vi "Temperature Decline Tester.vi"() -> ()   [LabVIEW 2023]
uses:
  Type Definitions/HEWH Output Information.ctl
  Type Definitions/HEWH Draw Pattern Setup.ctl
  Type Definitions/PRAT Test.ctl
  Utility/Save File/File Setup (Public)/Type Definition/Save File HEWH Heating Control Mode.ctl
  Support VIs/Draw Water Specific/Type Definitions/Terminate Draw Conditions.ctl
  Type Definitions/HEWH Start Conditions.ctl
  Support VIs/Draw Water Specific/Type Definitions/Check Special Condtions.ctl
  Support VIs/Draw Water Specific/Type Definitions/HEWH Special Condition Check.ctl
  Type Definitions/HEWH Draw Flag ENUM.ctl
  Type Definitions/HEWH Specific DAQ.ctl
  Type Definitions/HEWH Power Data.ctl
  Type Definitions/HEWH Power Elements.ctl
  Utility/Type Definitions/UTILITY Power Analyzer.ctl
  Drivers/Viasala Indigo 520/Type Definitions/Viasala Indigo 520 Data.ctl
  Drivers/Tidal Engineering/Type Definitions/Tenney Environmental Chamber Data.ctl
  Type Definitions/HEWH Calc and Calibration.ctl
  Utility/Save File/File Setup (Public)/Type Definition/Save File DOE LabView Program.ctl
  Custom Instrument Control/MW100/Type Definitions/Station ID Selector.ctl
  Range/Type Definitions/RANGE ANSI Rate.ctl
  Custom Instrument Control/MW100/Type Definitions/HEWH Module 4 Relay Status.ctl
  Drivers/Inficon Fusion Micro GC/Type Definitions/Inficon Data.ctl
  Drivers/Alicat Gas Meter Driver/Sub-VIs/Data Cluster.ctl
  Utility/Save File/File Setup.lvlib
panel:
  out "first_iteration":dbl
  out "Run_Timer":dbl
  out "Start Time":dbl
  out "Temp Decline Complete":bool
  in  "Use_Temp_Decline_Method":i16
  in  "Purge_Until_Cutout":i16
  out "prev_cycle_count_out":i32
  out "show_trigger (Debug)":u16
  in  "TC Tree (AVG)":dbl
  in  "stop":bool
  in  "Draw Count":i32
  out "max_temp":dbl
  out "Loop Counter":i32
  out "trigger":u8
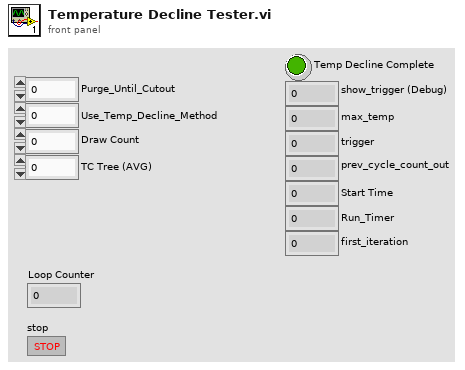
[diagram p1: front panel]
types:
  T1 = typedef "HEWH Output Information.ctl" = cluster{"Scan Rate Adjust":dbl, "Draw Count":i32, "Test Patten Setup":T2, "HEWH Specific DAQ":T10, "Test Output Data":cluster{"PreDraw Data Table":string[][], "Data Table":string[][], "MW100 TC Headers":string[]}, "Calc and Calibration":T16, "Current Draw Time":dbl, "LV Program":T17, "Station ID":T18, "Current Cond":T8, "Test Complete":bool, "ANSI Rate":T19, "Module 4 Relay Status":T20, "Inficon Data Output":T21, "Gas Measurements":cluster{"Gas Measurment Data -Alicat":T22, "Gas Measurment Data - Ritter":cluster{"Gas Flow Rate (L/hr)-Uncorrected":dbl, "Totalized Flow (L)--Uncorrected":dbl, "Gas Flow Rate (cuft/hr)-Uncorrected":dbl, "Totalized Flow (cuft)-Uncorrected":dbl, "Gas Temperature (F)":dbl, "Gas Pressure (in WC)":dbl, "Heise Barometric Pressure (inHG)":dbl, "STP Correction Factor":dbl, "Temp Correction Factor":dbl, "Pressure Correction Factor":dbl, "Water Vapor Pressure":dbl, "Gas Flow Rate (cuft/hr)-Corrected":dbl, "Totalized Flow (cuft)-Corrected":dbl}}}
  T2 = typedef "HEWH Draw Pattern Setup.ctl" = cluster{"Total Gallons Schedule":dbl[], "PRAT/RLT Sequence":T3[], "Current Sequence Index":i32}
  T3 = typedef "PRAT Test.ctl" = cluster{"Sequence #":dbl, "Cycles":i32, "Mode Setting":T4, "Flow Rate (GPM)":dbl, "Temperature (F)":dbl, "Reset Timer":bool, "Use Temp Decline Method":bool, "Terminate Condition":T5, "Condition Value #1":dbl, "UE":bool, "LE":bool, "Comp":bool, "Fan":bool, "Test End Time (Sec)":dbl, "Purge Until Cutout":bool, "Start Conditions":T6, "Condition Value #2":dbl, "Remove Power":bool, "Time":dbl, "Check Special Cond.":T7, "Condition#":T8, "Draw Flags":T9, "Data Processing Delay (FHD 15sec, UEF 5 Sec)":dbl, "Test Complete":bool, "User Setpoint":dbl, "Tank Setpoint":dbl}
  T4 = typedef "File Setup.lvlib/Save File HEWH Heating Control Mode.ctl" = string
  T5 = typedef "Terminate Draw Conditions.ctl" = enum16{"C1-Terminate Draw @ Gallon Mark", "C2-Special Last Draw (HU Test)", "C3-RTD Out <=", "C4-Mean Tank Temp <=", "C5-Decrease RTD Out (Deg F)", "C6-Time (Seconds)", "C7-Until Any Heat Source", "C8-Specific Heat Source", "C9-Do Nothing", "C10-Inlet Outlet RTD Temp Delta"}
  T6 = typedef "HEWH Start Conditions.ctl" = enum16{"Heat Source Cutout", "At Time (Seconds)", "Every X (Seconds)", "T2 >= X° Below Setpoint", "Seconds From Complete", "Wait for LE & Comp Cutout", "Wait for Comp Cutout", "Wait for LE Cutout", "Wait for UE Cutout", "Start Immediately"}
  T7 = typedef "Check Special Condtions.ctl" = enum16{"SC1-Do Nothing", "SC2-Check Heat Source (On-C2/Off-C1)", "SC3-Check Skip Condition", "SC4-Check Heat Source ON/Fail", "SC5-Keep Draw Valves Open", "SC6-Skip Purge"}
  T8 = typedef "HEWH Special Condition Check.ctl" = enum16{"N/A", "C1", "C2", "Reset/Fail", "Skip Draw Sequence"}
  T9 = typedef "HEWH Draw Flag ENUM.ctl" = enum16{"N/A", "None(0)", "Sml(1)", "Med(2)", "SmlMed(3)", "Lrg(4)", "SmlLrg(5)", "MedLrg(6)", "SmlMedLrg(7)"}
  T10 = typedef "HEWH Specific DAQ.ctl" = cluster{"HEWH Data":T11, "Flow Valve % Open":dbl, "Power State":T12, "Power Analyzer":T13, "Flow Valve uA Output":i32, "Gallons Start (Gal)":dbl, "PI Output":dbl, "Viasala Indigo 520 Data":T14, "Tenney Environmental Chamber Data Output":T15}
  T11 = typedef "HEWH Power Data.ctl" = cluster{"HEWH Standard":cluster{"Voltage (Volts)":dbl, "Current (Amps)":dbl, "Power (Watts)":dbl, "WattHours (Wh)":dbl, "TC Tree (AVG)":dbl, "Flow Rate (GPM)":dbl, "Gallons (Gal)":dbl, "RTD Out (Deg F)":dbl, "RTD In (Deg F)":dbl, "RTD Amb (Deg F)":dbl, "TC Down":dbl, "UE Event Lead":i32, "LE Event Lead":i32, "TC 8":dbl, "TC 9":dbl, "TC 10":dbl, "TC Tree Array (1-6)":dbl[], "TC 7":dbl, "PSI 1":dbl, "PSI 2":dbl, "PSI 3":dbl, "PSI 4":dbl, "Gas BTU":dbl, "Gas BTU/hr":dbl}, "PRAT":cluster{"Power (Watts) A":dbl, "Power (Watts) B":dbl, "Power (Watts) C":dbl, "Power (Watts) D":dbl, "TC1":dbl, "TC2":dbl, "TC3":dbl, "TC4":dbl, "WattHours (Wh) A":dbl, "WattHours (Wh) B":dbl, "WattHours (Wh) C":dbl, "WattHours (Wh) D":dbl, "Ambient":dbl, "Extra Temp":dbl}, "Additional Power Data":cluster{"Vthd":dbl, "Frequency (Hz)":dbl, "Apparent Power (VA)":dbl, "Power Factor":dbl, "Current Crest Factor":dbl, "Voltage Crest Factor":dbl, "Integration Time (sec)":dbl}}
  T12 = typedef "HEWH Power Elements.ctl" = cluster{"UE":bool, "LE":bool, "COMP":bool, "FANS":bool}
  T13 = typedef "UTILITY Power Analyzer.ctl" = enum16{"", "APLUS", "WT210", "WT500", "WT300", "OSI", "Debug", "WT230", "WT300_1", "WT300_2"}
  T14 = typedef "Viasala Indigo 520 Data.ctl" = cluster{"Temperature Probe 1":dbl, "Humidity Probe 1":dbl, "Temperature Probe 2":dbl, "Humidity Probe 2":dbl}
  T15 = typedef "Tenney Environmental Chamber Data.ctl" = cluster{"Temperature Setpoint":dbl, "Temperature Process Variable":dbl, "Humidity Setpoint":dbl, "Humidity Process Variable":dbl, "Frequency Setpoint":dbl, "Frequency Process Variable":dbl, "Chamber Status (ON/OFF)":string}
  T16 = typedef "HEWH Calc and Calibration.ctl" = cluster{"Mean SD Var Max Min Array":string[][], "Draw Statistics (DBL)":dbl[][], "Calibration Coefficients DBL":dbl[][], "Start Gallons":dbl, "Starting Temp Decline":dbl, "K-Factor (Temperature)":dbl, "All Draw Stats":string[][], "RTD Terminate Value":dbl, "K-Factor (Flow)":dbl, "Intellifaucet Type":string, "Thermal Stabil Array":dbl[][], "Gas Thermal Stabil Complete":bool, "Therm Reset Cmpt 1":bool, "Therm Reset Cmpt 2":bool, "Last Flow Rate (Therm)":dbl, "State":enum16{"State 0", "State 1", "State 2", "State 3", "State 4", "State 5", "State 6"}, "Gas Thermal Time":dbl, "Target Rate (Thermal)":dbl, "Thermal - Final":dbl[][], "State5 Gal Water":dbl, "State 5 Gal Gas":dbl, "Intellif Open < 1":dbl, "Intellif Open < 1.7":dbl, "Intellif Open < 2.2":dbl, "Intellif Open > 2.2":dbl, "End of Draw\nComparison":bool[][], "Temperature Decline Method":cluster{"Previous Cycle Count":i32, "Previous Max Temp In":dbl, "Previous Trigger In":u8, "Start Timer":dbl, "first_iteration":dbl}}
  T17 = typedef "File Setup.lvlib/Save File DOE LabView Program.ctl" = enum16{"No Name Found", "DOE Stand", "Dishwasher Kitchen", "Portable Stand", "HEWH", "Dryer", "Dryer WILT", "HCC", "PRAT", "HEWH RLT", "Refrigeration", "Gas Water Heater"}
  T18 = typedef "Station ID Selector.ctl" = enum16{"", "A", "B", "C", "D", "Global"}
  T19 = typedef "RANGE ANSI Rate.ctl" = cluster{"Array 1":dbl[], "Array 3":dbl[], "Array 2":dbl[], "Start ANSI":bool, "ANSI Start Time":dbl, "Restart ANSI":bool, "15 Min ANSI Avg (BTU/hr)":dbl, "20 Min ANSI Avg (BTU/hr)":dbl, "25 Min ANSI Avg (BTU/hr)":dbl, "Absolute Pressure":dbl, "Gas Temperature":dbl, "Volumetric Flow Rate":dbl, "Mass Flow Rate":dbl, "Array 4":dbl[], "Array 5":dbl[], "Gas Rate":dbl, "15 Min Pres Avg (PSIA)":dbl, "20 Min Pres Avg (PSIA)":dbl, "25 Min Pres Avg (PSIA)":dbl, "15 Min Temp Avg (°F) ":dbl, "20 Min Temp Avg (°F)":dbl, "25 Min Temp Avg (°F)":dbl, "15 Min Uncorrected Avg (CFH)":dbl, "20 Min Uncorrected Avg (CFH)":dbl, "25 Min Uncorrected Avg (CFH)":dbl, "15 Min Corrected Avg (SCFH)":dbl, "20 Min Corrected Avg (SCFH)":dbl, "25 Min Corrected Avg (SCFH)":dbl, "15 Min Complete":bool, "20 Min Complete":bool, "25 Min Complete":bool, "Heating Value (BTU/ft³)":dbl, "CO CO2 15 Min":string[][], "CO CO2 20 Min":string[][], "CO CO2 25 Min":string[][], "CO CO2 Real Time":string[][]}
  T20 = typedef "HEWH Module 4 Relay Status.ctl" = cluster{"INTELLIFAUCET TEMP(T)/FLOW(F) (CH 041)":bool, "INTELLIFAUCET READY (CH 042)":bool, "INTELLIFAUCET START (CH 043)":bool, "INTELLIFAUCET STOP (CH 044)":bool, "MAIN POWER RELAY (CH 047)":bool, "NOT USED (CH 045)":bool, "NOT USED (CH 046)":bool, "PURGE VALVE RELAY (CH 048)":bool, "OUTLET VALVE RELAY (CH 049)":bool, "INLET VALVE RELAY (CH 050)":bool, "Intellifaucet (% Open)":dbl, "Proportioning Valve (%Open)":dbl, "Intellifaucet Temp Setpoint (F)":dbl}
  T21 = typedef "Inficon Data.ctl" = cluster{"Gross Heating Value, Vol (Real, Dry)":dbl, "Nitrogen Component Normalized Mole % (Dry)":dbl, "Methane Component Normalized Mole % (Dry)":dbl, "Carbon Dioxide Component Normalized Mole % (Dry)":dbl, "Ethane Component Normalized Mole % (Dry)":dbl, "Propane Component Normalized Mole % (Dry)":dbl, "i-Pentane Component Normalized Mole % (Dry)":dbl, "i-Butane Component Normalized Mole % (Dry)":dbl, "n-Butane Component Normalized Mole % (Dry)":dbl, "n-Pentane Component Normalized Mole % (Dry)":dbl, "Hexane Component Normalized Mole % (Dry)":dbl, "Heptane Component Normalized Mole % (Dry)":dbl, "Gross Wobbe Index, Real(Dry)":dbl, "Relative Density, Real(Dry)":dbl, "Propylene Component Normalized Mole % (Dry)":dbl, "C4 Olefins Component Normalized Mole % (Dry)":dbl, "Water Component Normalized Mole % (Dry)":dbl, "Gross Heating Value, Vol (Real, Sat)":dbl}
  T22 = typedef "Data Cluster.ctl" = cluster{"Absolute Pressure":dbl, "Gauge/Diff. Pressure":dbl, "Barometric Pressure":dbl, "Temperature":dbl, "Volumetric Flow":dbl, "Mass Flow":dbl, "Setpoint":dbl, "Valve Drive":dbl, "Totalizer":dbl, "[hr]":dbl, "[min]":dbl, "[sec]":dbl, "Totalizer Average Flow":dbl, "Totalizer Peak Flow":dbl, "Gas selected":string}
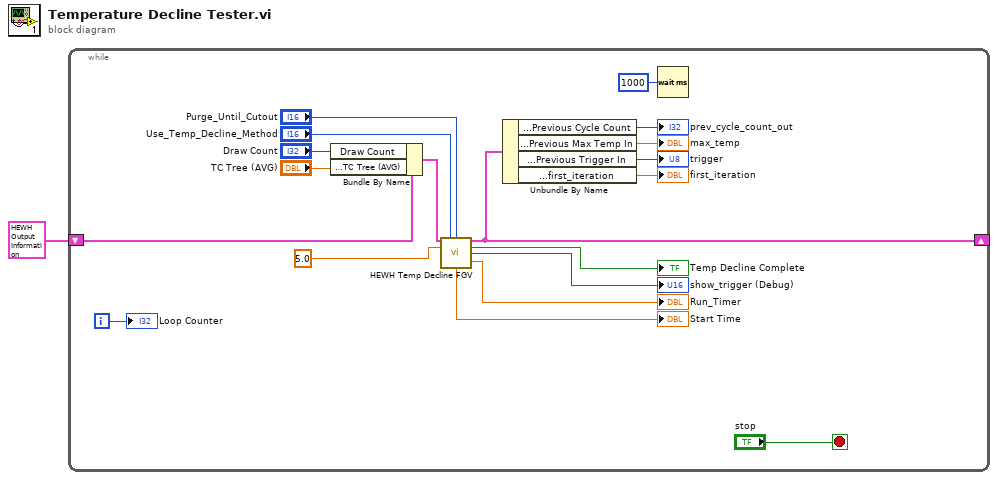
[diagram p0: block diagram]
diagram:
  n1 = while {
    shift-right: [w11] -> _
    shift-left: T1 {"Scan Rate Adjust"=0.0, "Draw Count"=0, "Test Patten Setup"={"Total Gallons Schedule"=[], "PRAT/RLT Sequence"=[{"Sequence #"=1.0, "Cycles"=35, "Mode Setting"="", "Flow Rate (GPM)"=0.0, "Temperature (F)"=0.0, "Reset Timer"=FALSE, "Use Temp Decline Method"=FALSE, "Terminate Condition"=enum."C1-Terminate Draw @ Gallon Mark", "Condition Value #1"=0.0, "UE"=FALSE, "LE"=FALSE, "Comp"=FALSE, "Fan"=FALSE, "Test End Time (Sec)"=0.0, "Purge Until Cutout"=FALSE, "Start Conditions"=enum."Heat Source Cutout", "Condition Value #2"=0.0, "Remove Power"=FALSE, "Time"=0.0, "Check Special Cond."=enum."SC1-Do Nothing", "Condition#"=enum."C1", "Draw Flags"=enum."N/A", "Data Processing Delay (FHD 15sec, UEF 5 Sec)"=0.0, "Test Complete"=FALSE, "User Setpoint"=0.0, "Tank Setpoint"=0.0}, {"Sequence #"=2.0, "Cycles"=15, "Mode Setting"="", "Flow Rate (GPM)"=0.0, "Temperature (F)"=0.0, "Reset Timer"=FALSE, "Use Temp Decline Method"=FALSE, "Terminate Condition"=enum."C1-Terminate Draw @ Gallon Mark", "Condition Value #1"=0.0, "UE"=FALSE, "LE"=FALSE, "Comp"=FALSE, "Fan"=FALSE, "Test End Time (Sec)"=0.0, "Purge Until Cutout"=FALSE, "Start Conditions"=enum."Heat Source Cutout", "Condition Value #2"=0.0, "Remove Power"=FALSE, "Time"=0.0, "Check Special Cond."=enum."SC1-Do Nothing", "Condition#"=enum."C1", "Draw Flags"=enum."N/A", "Data Processing Delay (FHD 15sec, UEF 5 Sec)"=0.0, "Test Complete"=FALSE, "User Setpoint"=0.0, "Tank Setpoint"=0.0}, {"Sequence #"=3.0, "Cycles"=35, "Mode Setting"="", "Flow Rate (GPM)"=0.0, "Temperature (F)"=0.0, "Reset Timer"=FALSE, "Use Temp Decline Method"=FALSE, "Terminate Condition"=enum."C1-Terminate Draw @ Gallon Mark", "Condition Value #1"=0.0, "UE"=FALSE, "LE"=FALSE, "Comp"=FALSE, "Fan"=FALSE, "Test End Time (Sec)"=0.0, "Purge Until Cutout"=FALSE, "Start Conditions"=enum."Heat Source Cutout", "Condition Value #2"=0.0, "Remove Power"=FALSE, "Time"=0.0, "Check Special Cond."=enum."SC1-Do Nothing", "Condition#"=enum."C1", "Draw Flags"=enum."N/A", "Data Processing Delay (FHD 15sec, UEF 5 Sec)"=0.0, "Test Complete"=FALSE, "User Setpoint"=0.0, "Tank Setpoint"=0.0}, {"Sequence #"=4.0, "Cycles"=15, "Mode Setting"="", "Flow Rate (GPM)"=0.0, "Temperature (F)"=0.0, "Reset Timer"=FALSE, "Use Temp Decline Method"=FALSE, "Terminate Condition"=enum."C1-Terminate Draw @ Gallon Mark", "Condition Value #1"=0.0, "UE"=FALSE, "LE"=FALSE, "Comp"=FALSE, "Fan"=FALSE, "Test End Time (Sec)"=0.0, "Purge Until Cutout"=FALSE, "Start Conditions"=enum."Heat Source Cutout", "Condition Value #2"=0.0, "Remove Power"=FALSE, "Time"=0.0, "Check Special Cond."=enum."SC1-Do Nothing", "Condition#"=enum."C1", "Draw Flags"=enum."N/A", "Data Processing Delay (FHD 15sec, UEF 5 Sec)"=0.0, "Test Complete"=FALSE, "User Setpoint"=0.0, "Tank Setpoint"=0.0}, {"Sequence #"=5.0, "Cycles"=35, "Mode Setting"="", "Flow Rate (GPM)"=0.0, "Temperature (F)"=0.0, "Reset Timer"=FALSE, "Use Temp Decline Method"=FALSE, "Terminate Condition"=enum."C1-Terminate Draw @ Gallon Mark", "Condition Value #1"=0.0, "UE"=FALSE, "LE"=FALSE, "Comp"=FALSE, "Fan"=FALSE, "Test End Time (Sec)"=0.0, "Purge Until Cutout"=FALSE, "Start Conditions"=enum."Heat Source Cutout", "Condition Value #2"=0.0, "Remove Power"=FALSE, "Time"=0.0, "Check Special Cond."=enum."SC1-Do Nothing", "Condition#"=enum."C1", "Draw Flags"=enum."N/A", "Data Processing Delay (FHD 15sec, UEF 5 Sec)"=0.0, "Test Complete"=FALSE, "User Setpoint"=0.0, "Tank Setpoint"=0.0}, {"Sequence #"=6.0, "Cycles"=15, "Mode Setting"="", "Flow Rate (GPM)"=0.0, "Temperature (F)"=0.0, "Reset Timer"=FALSE, "Use Temp Decline Method"=FALSE, "Terminate Condition"=enum."C1-Terminate Draw @ Gallon Mark", "Condition Value #1"=0.0, "UE"=FALSE, "LE"=FALSE, "Comp"=FALSE, "Fan"=FALSE, "Test End Time (Sec)"=0.0, "Purge Until Cutout"=FALSE, "Start Conditions"=enum."Heat Source Cutout", "Condition Value #2"=0.0, "Remove Power"=FALSE, "Time"=0.0, "Check Special Cond."=enum."SC1-Do Nothing", "Condition#"=enum."C1", "Draw Flags"=enum."N/A", "Data Processing Delay (FHD 15sec, UEF 5 Sec)"=0.0, "Test Complete"=FALSE, "User Setpoint"=0.0, "Tank Setpoint"=0.0}, {"Sequence #"=7.0, "Cycles"=35, "Mode Setting"="", "Flow Rate (GPM)"=0.0, "Temperature (F)"=0.0, "Reset Timer"=FALSE, "Use Temp Decline Method"=FALSE, "Terminate Condition"=enum."C1-Terminate Draw @ Gallon Mark", "Condition Value #1"=0.0, "UE"=FALSE, "LE"=FALSE, "Comp"=FALSE, "Fan"=FALSE, "Test End Time (Sec)"=0.0, "Purge Until Cutout"=FALSE, "Start Conditions"=enum."Heat Source Cutout", "Condition Value #2"=0.0, "Remove Power"=FALSE, "Time"=0.0, "Check Special Cond."=enum."SC1-Do Nothing", "Condition#"=enum."C1", "Draw Flags"=enum."N/A", "Data Processing Delay (FHD 15sec, UEF 5 Sec)"=0.0, "Test Complete"=FALSE, "User Setpoint"=0.0, "Tank Setpoint"=0.0}, {"Sequence #"=8.0, "Cycles"=15, "Mode Setting"="", "Flow Rate (GPM)"=0.0, "Temperature (F)"=0.0, "Reset Timer"=FALSE, "Use Temp Decline Method"=FALSE, "Terminate Condition"=enum."C1-Terminate Draw @ Gallon Mark", "Condition Value #1"=0.0, "UE"=FALSE, "LE"=FALSE, "Comp"=FALSE, "Fan"=FALSE, "Test End Time (Sec)"=0.0, "Purge Until Cutout"=FALSE, "Start Conditions"=enum."Heat Source Cutout", "Condition Value #2"=0.0, "Remove Power"=FALSE, "Time"=0.0, "Check Special Cond."=enum."SC1-Do Nothing", "Condition#"=enum."C1", "Draw Flags"=enum."N/A", "Data Processing Delay (FHD 15sec, UEF 5 Sec)"=0.0, "Test Complete"=FALSE, "User Setpoint"=0.0, "Tank Setpoint"=0.0}], "Current Sequence Index"=0}, "HEWH Specific DAQ"={"HEWH Data"={"HEWH Standard"={"Voltage (Volts)"=0.0, "Current (Amps)"=0.0, "Power (Watts)"=0.0, "WattHours (Wh)"=0.0, "TC Tree (AVG)"=0.0, "Flow Rate (GPM)"=0.0, "Gallons (Gal)"=0.0, "RTD Out (Deg F)"=0.0, "RTD In (Deg F)"=0.0, "RTD Amb (Deg F)"=0.0, "TC Down"=0.0, "UE Event Lead"=0, "LE Event Lead"=0, "TC 8"=0.0, "TC 9"=0.0, "TC 10"=0.0, "TC Tree Array (1-6)"=[], "TC 7"=0.0, "PSI 1"=0.0, "PSI 2"=0.0, "PSI 3"=0.0, "PSI 4"=0.0, "Gas BTU"=0.0, "Gas BTU/hr"=0.0}, "PRAT"={"Power (Watts) A"=0.0, "Power (Watts) B"=0.0, "Power (Watts) C"=0.0, "Power (Watts) D"=0.0, "TC1"=0.0, "TC2"=0.0, "TC3"=0.0, "TC4"=0.0, "WattHours (Wh) A"=0.0, "WattHours (Wh) B"=0.0, "WattHours (Wh) C"=0.0, "WattHours (Wh) D"=0.0, "Ambient"=0.0, "Extra Temp"=0.0}, "Additional Power Data"={"Vthd"=0.0, "Frequency (Hz)"=0.0, "Apparent Power (VA)"=0.0, "Power Factor"=0.0, "Current Crest Factor"=0.0, "Voltage Crest Factor"=0.0, "Integration Time (sec)"=0.0}}, "Flow Valve % Open"=0.0, "Power State"={"UE"=FALSE, "LE"=FALSE, "COMP"=FALSE, "FANS"=FALSE}, "Power Analyzer"=enum."APLUS", "Flow Valve uA Output"=0, "Gallons Start (Gal)"=0.0, "PI Output"=0.0, "Viasala Indigo 520 Data"={"Temperature Probe 1"=0.0, "Humidity Probe 1"=0.0, "Temperature Probe 2"=0.0, "Humidity Probe 2"=0.0}, "Tenney Environmental Chamber Data Output"={"Temperature Setpoint"=0.0, "Temperature Process Variable"=0.0, "Humidity Setpoint"=0.0, "Humidity Process Variable"=0.0, "Frequency Setpoint"=0.0, "Frequency Process Variable"=0.0, "Chamber Status (ON/OFF)"=""}}, "Test Output Data"={"PreDraw Data Table"=[], "Data Table"=[], "MW100 TC Headers"=[]}, "Calc and Calibration"={"Mean SD Var Max Min Array"=[], "Draw Statistics (DBL)"=[], "Calibration Coefficients DBL"=[], "Start Gallons"=0.0, "Starting Temp Decline"=0.0, "K-Factor (Temperature)"=0.0, "All Draw Stats"=[], "RTD Terminate Value"=0.0, "K-Factor (Flow)"=0.0, "Intellifaucet Type"="", "Thermal Stabil Array"=[], "Gas Thermal Stabil Complete"=FALSE, "Therm Reset Cmpt 1"=FALSE, "Therm Reset Cmpt 2"=FALSE, "Last Flow Rate (Therm)"=0.0, "State"=enum."State 1", "Gas Thermal Time"=0.0, "Target Rate (Thermal)"=0.0, "Thermal - Final"=[], "State5 Gal Water"=0.0, "State 5 Gal Gas"=0.0, "Intellif Open < 1"=0.0, "Intellif Open < 1.7"=0.0, "Intellif Open < 2.2"=0.0, "Intellif Open > 2.2"=0.0, "End of Draw\nComparison"=[], "Temperature Decline Method"={"Previous Cycle Count"=0, "Previous Max Temp In"=0.0, "Previous Trigger In"=0, "Start Timer"=0.0, "first_iteration"=0.0}}, "Current Draw Time"=0.0, "LV Program"=enum."HEWH", "Station ID"=enum."A", "Current Cond"=enum."N/A", "Test Complete"=FALSE, "ANSI Rate"={"Array 1"=[], "Array 3"=[], "Array 2"=[], "Start ANSI"=FALSE, "ANSI Start Time"=0.0, "Restart ANSI"=FALSE, "15 Min ANSI Avg (BTU/hr)"=0.0, "20 Min ANSI Avg (BTU/hr)"=0.0, "25 Min ANSI Avg (BTU/hr)"=0.0, "Absolute Pressure"=0.0, "Gas Temperature"=0.0, "Volumetric Flow Rate"=0.0, "Mass Flow Rate"=0.0, "Array 4"=[], "Array 5"=[], "Gas Rate"=0.0, "15 Min Pres Avg (PSIA)"=0.0, "20 Min Pres Avg (PSIA)"=0.0, "25 Min Pres Avg (PSIA)"=0.0, "15 Min Temp Avg (°F) "=0.0, "20 Min Temp Avg (°F)"=0.0, "25 Min Temp Avg (°F)"=0.0, "15 Min Uncorrected Avg (CFH)"=0.0, "20 Min Uncorrected Avg (CFH)"=0.0, "25 Min Uncorrected Avg (CFH)"=0.0, "15 Min Corrected Avg (SCFH)"=0.0, "20 Min Corrected Avg (SCFH)"=0.0, "25 Min Corrected Avg (SCFH)"=0.0, "15 Min Complete"=FALSE, "20 Min Complete"=FALSE, "25 Min Complete"=FALSE, "Heating Value (BTU/ft³)"=0.0, "CO CO2 15 Min"=[], "CO CO2 20 Min"=[], "CO CO2 25 Min"=[], "CO CO2 Real Time"=[]}, "Module 4 Relay Status"={"INTELLIFAUCET TEMP(T)/FLOW(F) (CH 041)"=FALSE, "INTELLIFAUCET READY (CH 042)"=FALSE, "INTELLIFAUCET START (CH 043)"=FALSE, "INTELLIFAUCET STOP (CH 044)"=FALSE, "MAIN POWER RELAY (CH 047)"=FALSE, "NOT USED (CH 045)"=FALSE, "NOT USED (CH 046)"=FALSE, "PURGE VALVE RELAY (CH 048)"=FALSE, "OUTLET VALVE RELAY (CH 049)"=FALSE, "INLET VALVE RELAY (CH 050)"=FALSE, "Intellifaucet (% Open)"=0.0, "Proportioning Valve (%Open)"=0.0, "Intellifaucet Temp Setpoint (F)"=0.0}, "Inficon Data Output"={"Gross Heating Value, Vol (Real, Dry)"=1067.4462890625, "Nitrogen Component Normalized Mole % (Dry)"=0.0, "Methane Component Normalized Mole % (Dry)"=92.87550354003906, "Carbon Dioxide Component Normalized Mole % (Dry)"=0.1941000074148178, "Ethane Component Normalized Mole % (Dry)"=6.454999923706055, "Propane Component Normalized Mole % (Dry)"=0.3865000009536743, "i-Pentane Component Normalized Mole % (Dry)"=0.007799999788403511, "i-Butane Component Normalized Mole % (Dry)"=0.03880000114440918, "n-Butane Component Normalized Mole % (Dry)"=0.03819999843835831, "n-Pentane Component Normalized Mole % (Dry)"=0.004100000020116568, "Hexane Component Normalized Mole % (Dry)"=0.0, "Heptane Component Normalized Mole % (Dry)"=0.0, "Gross Wobbe Index, Real(Dry)"=1385.8905029296875, "Relative Density, Real(Dry)"=0.5932452082633972, "Propylene Component Normalized Mole % (Dry)"=0.0, "C4 Olefins Component Normalized Mole % (Dry)"=0.0, "Water Component Normalized Mole % (Dry)"=0.0, "Gross Heating Value, Vol (Real, Sat)"=0.0}, "Gas Measurements"={"Gas Measurment Data -Alicat"={"Absolute Pressure"=0.0, "Gauge/Diff. Pressure"=0.0, "Barometric Pressure"=0.0, "Temperature"=0.0, "Volumetric Flow"=0.0, "Mass Flow"=0.0, "Setpoint"=0.0, "Valve Drive"=0.0, "Totalizer"=0.0, "[hr]"=0.0, "[min]"=0.0, "[sec]"=0.0, "Totalizer Average Flow"=0.0, "Totalizer Peak Flow"=0.0, "Gas selected"=""}, "Gas Measurment Data - Ritter"={"Gas Flow Rate (L/hr)-Uncorrected"=0.0, "Totalized Flow (L)--Uncorrected"=0.0, "Gas Flow Rate (cuft/hr)-Uncorrected"=0.0, "Totalized Flow (cuft)-Uncorrected"=0.0, "Gas Temperature (F)"=0.0, "Gas Pressure (in WC)"=0.0, "Heise Barometric Pressure (inHG)"=0.0, "STP Correction Factor"=0.0, "Temp Correction Factor"=0.0, "Pressure Correction Factor"=0.0, "Water Vapor Pressure"=0.0, "Gas Flow Rate (cuft/hr)-Corrected"=0.0, "Totalized Flow (cuft)-Corrected"=0.0}}} ("Core HEWH Data IN") -> [w17]
    i -> [w20]
    stop <- "stop" stop-if-true
    n2 = Bundle By Name(cluster=w17, "Draw Count"="Draw Count", "HEWH Specific DAQ.HEWH Data.HEWH Standard.TC Tree (AVG)"="TC Tree (AVG)") -> (w16:T1)
    n3 = call "HEWH Temp Decline FGV.vi"("Core HEWH Data IN"=w16, "Use_Temp_Decline_Method"="Use_Temp_Decline_Method", "Purge_Until_Cutout"="Purge_Until_Cutout", "decrement_threshold"=5.0) -> ("Core HEWH Data Out"=w11:T1, "Temp Decline Complete"=→"Temp Decline Complete":bool, "show_trigger (Debug)"=→"show_trigger (Debug)":u16, "Start Time"=→"Start Time":dbl, "Run_Timer"=→"Run_Timer":dbl)  [unwired: 6 in, 1 out]
    n4 = Unbundle By Name(w11) -> ("Calc and Calibration.Temperature Decline Method.Previous Cycle Count"=→"prev_cycle_count_out":i32, "Calc and Calibration.Temperature Decline Method.Previous Max Temp In"=→"max_temp":dbl, "Calc and Calibration.Temperature Decline Method.Previous Trigger In"=→"trigger":u8, "Calc and Calibration.Temperature Decline Method.first_iteration"=→"first_iteration":dbl)
    n5 = Wait (ms)(milliseconds to wait=u32 1000) -> ()  [unwired: 1 out]
    "Loop Counter" <- w20
  }
